vi "Set Condition for Waveform Stream (In Range DBL).vi"(7 "invert range check? (F)":bool, 8 "error in (no error)":errorcluster, 9 "low limit":dbl, 10 "high limit":dbl, 11 "WaveformStreamSpecification in":T1) -> (0 "error out":errorcluster, 3 "WaveformStreamSpecification out":T1)   [LabVIEW 2020, in "NI_VS Waveform Streaming Interface.lvlib"]
doc: "Defines the condition under which NI VeriStand streams waveform data to a host computer."
uses:
  <vilib>/NI VeriStand/Execution/WaveformStreaming/NI_VS Waveform Streaming Interface.lvlib
  <vilib>/NI VeriStand/Execution/WaveformStreaming/WaveformStreamSpecification.ctl
  NationalInstruments.VeriStand.ClientAPI
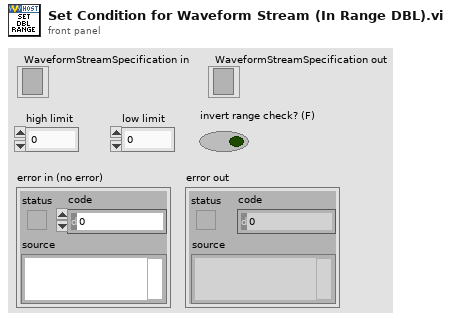
[diagram p1: front panel]
types:
  T1 = typedef "NI_VS Waveform Streaming Interface.lvlib/WaveformStreamSpecification.ctl" = refnum<k24>
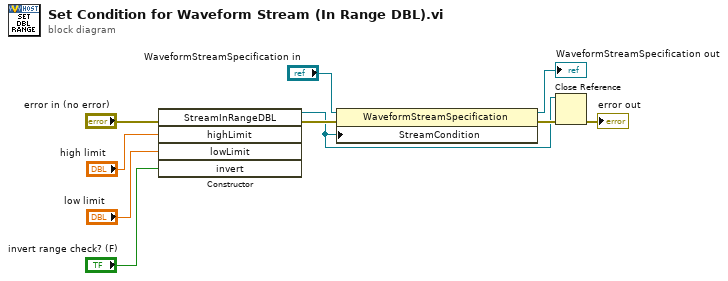
[diagram p0: block diagram]
diagram:
  n1 = constructor class="StreamInRangeDBL"(error in="error in (no error)", "highLimit"="high limit", "lowLimit"="low limit", "invert"="invert range check? (F)") -> (reference out=w4:refnum<k24>, error out=w6:errorcluster)  [unwired: 2 in, 4 out]
  n2 = property class="WaveformStreamSpecification"(reference="WaveformStreamSpecification in", error in=w6, "StreamCondition"=w4) -> (reference out=→"WaveformStreamSpecification out":T1, error out=w5:errorcluster)
  n3 = Close Reference(reference=w4, error in (no error)=w5) -> (error out=→"error out":errorcluster)
